vi "Check Auth.vi"(6 "Google OAuth":refnum<class "OAuth2.lvclass">, 7 "Authorization in":refnum<class "Authorization.lvclass">, 8 "error in (no error)":errorcluster, 11 "Gmail in":refnum<class "Gmail.lvclass">) -> (0 "error out":errorcluster, 3 "Gmail out":refnum<class "Gmail.lvclass">, 5 "Authorization":refnum<class "Authorization.lvclass">)   [LabVIEW 2020, in "Gmail API.lvlib" / "Gmail.lvclass"]
uses:
  Gmail.lvclass
  <vilib>/IlluminatedG/IG HTTP Utils/OAuth2/Authorization/Authorization.lvclass
  OAuth2/OAuth2.lvclass
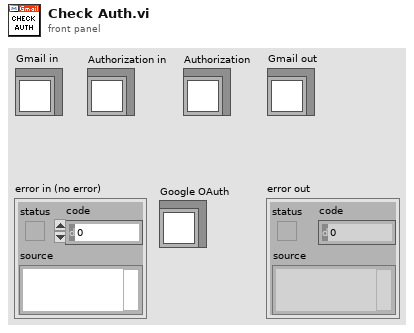
[diagram p1: front panel]
types:
  T1 = typedef "OAuth2.lvlib/Expiry.ctl" = enum16{"Unknown", "Expired", "Good"}
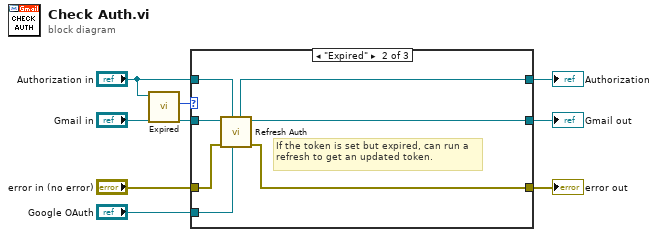
[diagram p0: block diagram]
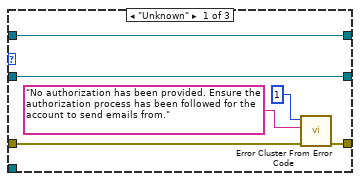
[diagram p2: hidden frame]
diagram:
  n1 = call <vilib>:"Expired.vi"("Authorization in"="Authorization in") -> ("Expiry"=w8:T1)  [unwired: 10 in]
  n2 = case shown="\"Expired\"" w8 {
    tunnel: "Authorization in" -> [w11 w20 w22]
    tunnel: "Gmail in" -> [w9 w21 w23]
    tunnel: "error in (no error)" -> [w14 w17 w24]
    tunnel: "Google OAuth" -> [_ w15 _]
    tunnel: [w11 w19 w22] -> w3
    tunnel: [w9 w18 w23] -> w2
    tunnel: [w10 w16 w24] -> w1
    frame "Unknown" {
      n3 = call <vilib>:"Error Cluster From Error Code.vi"("error in (no error)"=w14, "error message (\"\")"="No authorization has been provided. Ensure the authorization process has been followed for the account to send emails from." ("error message (\"\")"), "error code (0)"=1) -> ("error out"=w10:errorcluster)  [unwired: 6 in]
    }
    frame "Expired" {
      # "If the token is set but expired, can run a refresh to get an updated token."
      n4 = call "Refresh Auth.vi"("Google OAuth"=w15, "Authorization in"=w20, "error in (no error)"=w17, "Gmail in"=w21) -> ("error out"=w16:errorcluster, "Gmail out"=w18:refnum<class "Gmail.lvclass">, "Authorization"=w19:refnum<class "Authorization.lvclass">)  [unwired: 5 in]
    }
    frame "Good" {
    }
  }
  "error out" <- w1
  "Gmail out" <- w2
  "Authorization" <- w3
